vi "Get Master and Local Mod IOVs.vi"(8 "error in (no error)":errorcluster, 11 "IOV Engine in":refnum<k21>="ni.var.io:/") -> (0 "error IO":errorcluster, 1 "All Masters":refnum<k21>[](array[refnum]), 2 "All Local Mods":refnum<k21>[](array[refnum]), 3 "Local UDV Container":refnum<k21>[](array[refnum]))   [LabVIEW 2016, in "Scan Engine Custom Device.lvlib"]
uses:
  Scan Engine Custom Device.lvlib
  <resource>/objmgr/ni.var.rc
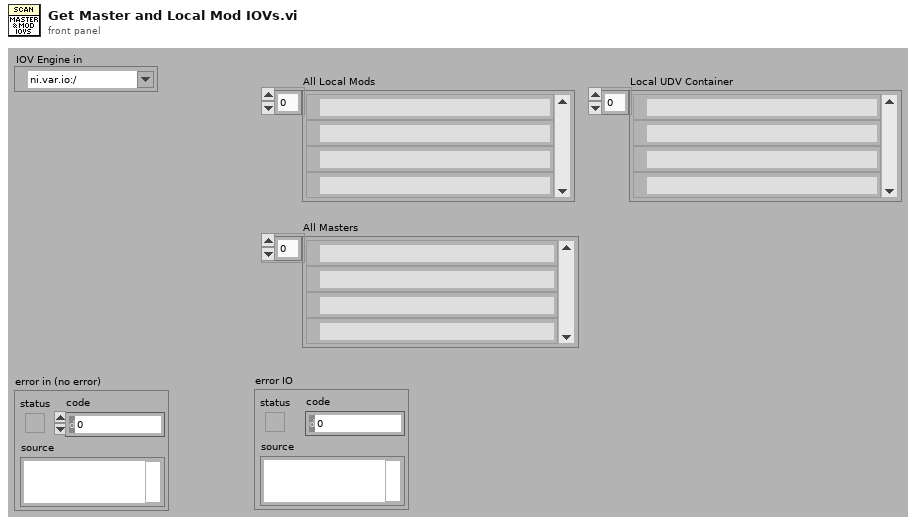
[diagram p1: front panel]
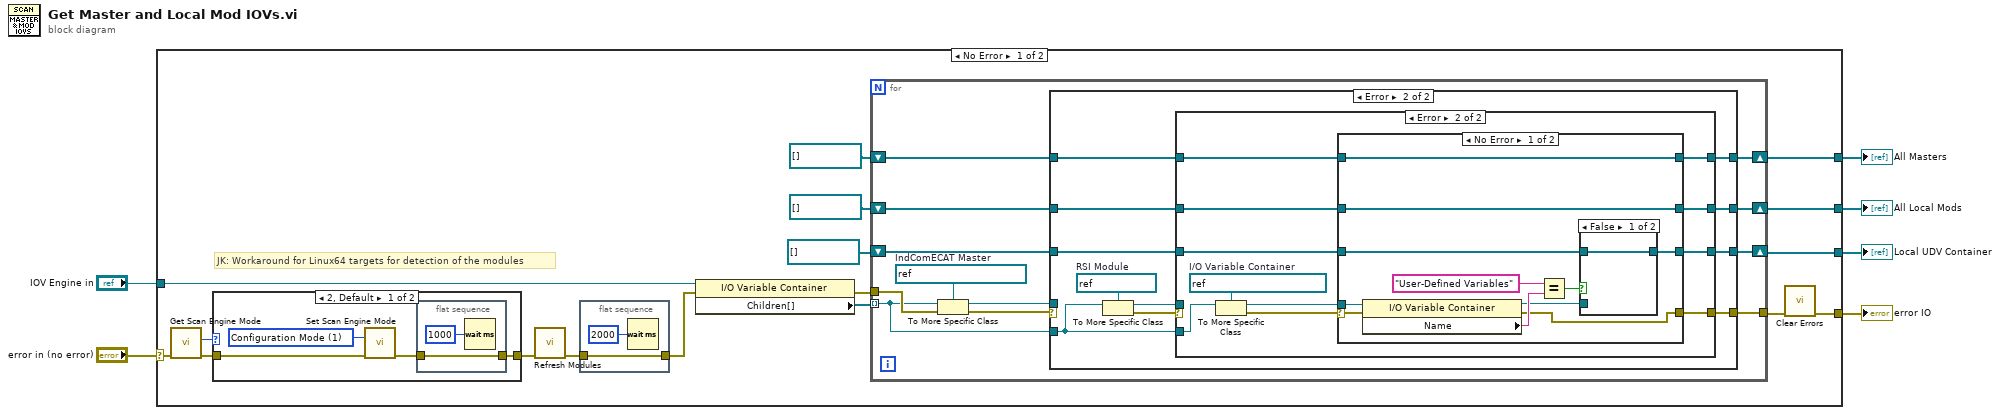
[diagram p0: block diagram]
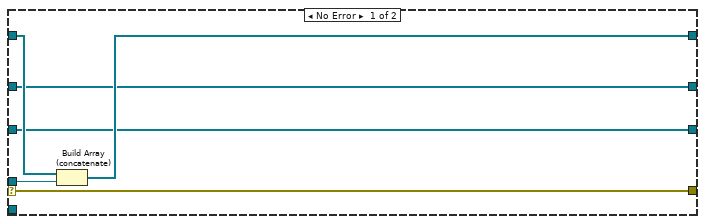
[diagram p3: hidden frame]
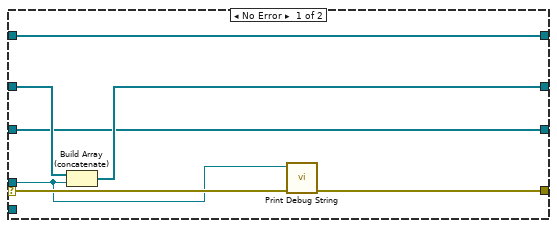
[diagram p4: hidden frame]
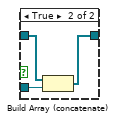
[diagram p5: hidden frame]
diagram:
  n1 = case shown="No Error" "error in (no error)" {
    selector: "error in (no error)" -> [w9 w99]
    tunnel: [w23 w99] -> w6
    tunnel: [w20 _] -> w5
    tunnel: "IOV Engine in" -> [w17 _]
    tunnel: [w15 _] -> w2
    tunnel: [w13 _] -> w1
    frame No Error {
      # "JK: Workaround for Linux64 targets for detection of the modules"
      n2 = call <vilib>:"Get Scan Engine Mode.vi"("error in (no error)"=w9) -> ("error out"=w11:errorcluster, "mode"=w10:i32)  [unwired: 9 in]
      n3 = case shown="2, Default" w10 {
        tunnel: w11 -> [w28 w32]
        tunnel: [w27 w32] -> w12
        frame 2, Default {
          w29 = 1 items=["Configuration Mode"=1, "Active Mode"=2] ("mode (Active Mode)")
          n4 = call <vilib>:"Set Scan Engine Mode.vi"("mode (Active Mode)"=w29, "error in (no error)"=w28) -> ("error out"=w26:errorcluster)  [unwired: 13 in]
          n5 = flat-sequence {
            tunnel: [w31] -> w27
            tunnel: w26 -> [w31]
            frame #0 {
              n6 = Wait (ms)(milliseconds to wait=u32 1000) -> ()  [unwired: 1 out]
            }
          }
        }
        frame 1 {
        }
      }
      n7 = call <vilib>:"Refresh Modules.vi"("error in (no error)"=w12) -> ("error out"=w8:errorcluster)  [unwired: 10 in]
      n8 = flat-sequence {
        tunnel: [w25] -> w7
        tunnel: w8 -> [w25]
        frame #0 {
          n9 = Wait (ms)(milliseconds to wait=u32 2000) -> ()  [unwired: 1 out]
        }
      }
      n10 = property class="I/O Variable Container"(reference=w17, error in=w7) -> (error out=w19:errorcluster, "Children[]"=w18:refnum<k21>[])  [unwired: 1 out]
      n11 = for {
        tunnel: w18 -> [w37] mode=indexing
        tunnel: w19 -> [w44]
        shift-right: [w40] -> w20
        shift-left: refnum<k21>[] [] -> [w39]
        tunnel: [w38] -> w22
        shift-right: [w35] -> w15
        shift-left: refnum<k21>[] [] -> [w36]
        shift-right: [w33] -> w13
        shift-left: refnum<k21>[] [] -> [w34]
        w43 = refnum<k21> refnum  # IndComECAT Master
        n12 = To More Specific Class(target class=w43, reference=w37, error in=w44) -> (specific class reference=w41:refnum<k21>, error out=w42:errorcluster)
        n13 = case shown="Error" w42 {
          selector: w42 -> [w48 _]
          tunnel: w41 -> [w45 _]
          tunnel: [w50 w55] -> w40
          tunnel: w39 -> [w49 w56]
          tunnel: [w48 w54] -> w38
          tunnel: w37 -> [_ w53]
          tunnel: w36 -> [w47 w58]
          tunnel: [w47 w57] -> w35
          tunnel: w34 -> [w46 w52]
          tunnel: [w46 w51] -> w33
          frame No Error {
            n14 = Build Array (concatenate)(w49, w45) -> (w50:refnum<k21>[])
          }
          frame Error {
            w61 = refnum<k21> refnum  # RSI Module
            n15 = To More Specific Class(target class=w61, reference=w53) -> (specific class reference=w59:refnum<k21>, error out=w60:errorcluster)  [unwired: 1 in]
            n16 = case shown="Error" w60 {
              tunnel: w59 -> [w62 _]
              selector: w60 -> [w63 _]
              tunnel: w58 -> [w68 w75]
              tunnel: [w67 w72] -> w57
              tunnel: w56 -> [w66 w74]
              tunnel: [w66 w73] -> w55
              tunnel: [w64 w69] -> w54
              tunnel: w53 -> [_ w78]
              tunnel: w52 -> [w65 w76]
              tunnel: [w65 w71] -> w51
              frame No Error {
                n17 = Build Array (concatenate)(w68, w62) -> (w67:refnum<k21>[])
                n18 = call "Print Debug String.vi"("error in"=w63, "String to write"=w62) -> ("error out"=w64:errorcluster)  [unwired: 8 in]
              }
              frame Error {
                w79 = refnum<k21> refnum  # I/O Variable Container
                n19 = To More Specific Class(target class=w79, reference=w78) -> (specific class reference=w70:refnum<k21>, error out=w77:errorcluster)  [unwired: 1 in]
                n20 = case shown="No Error" w77 {
                  selector: w77 -> [w88 w95]
                  tunnel: w76 -> [w82 w98]
                  tunnel: w75 -> [w89 w97]
                  tunnel: w74 -> [w90 w96]
                  tunnel: [w90 w96] -> w73
                  tunnel: [w89 w97] -> w72
                  tunnel: [w81 w98] -> w71
                  tunnel: w70 -> [w87 _]
                  tunnel: [w80 w95] -> w69
                  frame No Error {
                    n21 = property class="I/O Variable Container"(reference=w87, error in=w88) -> (reference out=w83:refnum<k21>, error out=w80:errorcluster, "Name"=w86:string)
                    n22 = Equal?(x="User-Defined Variables", y=w86) -> (x = y?=w84:bool)
                    n23 = case shown="False" w84 {
                      tunnel: w83 -> [_ w93]
                      tunnel: w82 -> [w91 w94]
                      tunnel: [w91 w92] -> w81
                      frame False {
                      }
                      frame True {
                        n24 = Build Array (concatenate)(w94, w93) -> (w92:refnum<k21>[])
                      }
                    }
                  }
                  frame Error {
                  }
                }
              }
            }
          }
        }
      }
      n25 = call <vilib>:"Clear Errors.vi"("error in (no error)"=w22) -> ("error out"=w23:errorcluster)  [unwired: 5 in, 1 out]
    }
    frame Error {
    }
  }
  "All Masters" <- w5
  "error IO" <- w6
  "All Local Mods" <- w2
  "Local UDV Container" <- w1
